vi "EoS.vi"() -> ()   [LabVIEW 2021]
panel:
  out "eV":dbl=0.016852039096730706
  in  "Volume":dbl=3e-29 format="%#_6em^3"
  in  "Pressure":dbl=3000000000.0 format="%#_6pPa"
  in  "Modulus":dbl=100000000000.0 format="%#_6pPa"
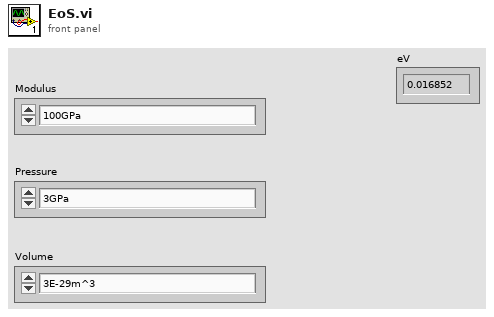
[diagram p1: front panel]
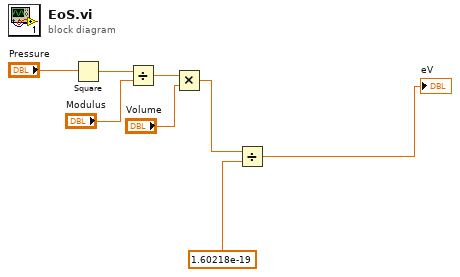
[diagram p0: block diagram]
diagram:
  n1 = Square(x="Pressure") -> (x^2=w7:dbl)
  n2 = Divide(x=w7, y="Modulus") -> (x/y=w5:dbl)
  n3 = Multiply(x=w5, y="Volume") -> (x*y=w3:dbl)
  n4 = Divide(x=w3, y=1.60218e-19) -> (x/y=→"eV":dbl)
